vi "6009 LV71.vi"() -> ()   [LabVIEW 2020]
uses:
  <vilib>/DAQmx/read.llb/DAQmx Read.vi
  <vilib>/DAQmx/read.llb/DAQmx Read (Analog 1D Wfm NChan NSamp).vi
  <vilib>/DAQmx/miscellaneous.llb/DAQmx Fill In Error Info.vi
panel:
  in  "Channel B":tag
  in  "Channel A":tag
  out "error out":errorcluster
  out "Origin ref":refnum<k7>
  in  "Show Origin":bool
  out "path":path
  out "OriginWks":refnum<k7>
  out "Samples in Buffer\n(Scan Backlog)":u32
  out "Reading Fast\nEnough?":bool
  in  "Read Wait (ms)":i32=200
  in  "Sampling Rate (Hz)":dbl(slide)=1000.0 min=100.0 max=20000.0 step=100.0 scale=100.0..20000.0 scale format="%#_4f"
  out "Buffer Size":dbl=1000.0
  out "Waveforms":waveform(dbl)[](graph)
  in  "stop":bool
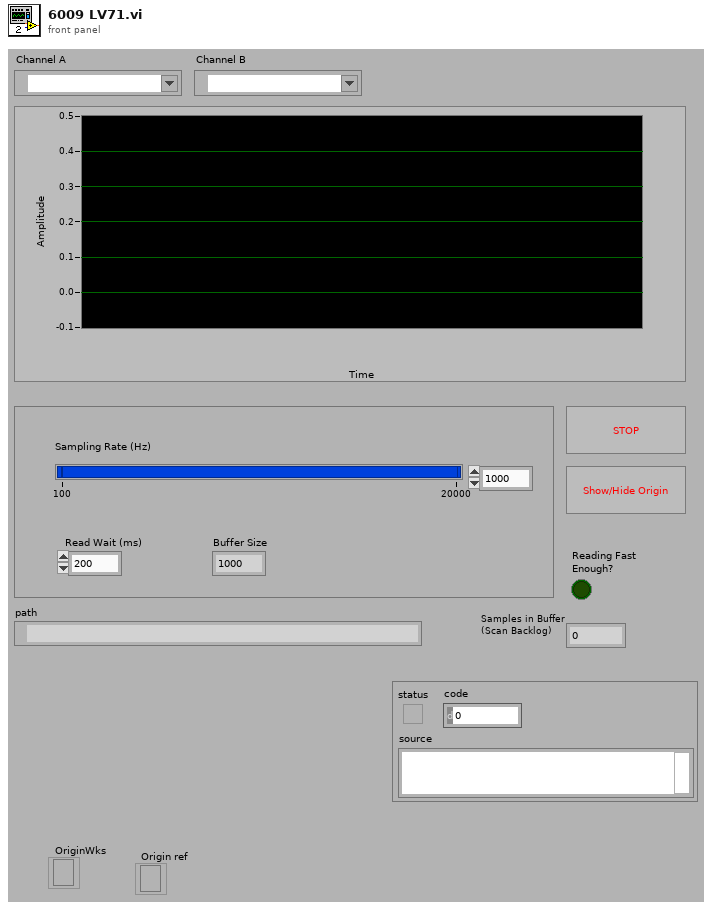
[diagram p1: front panel]
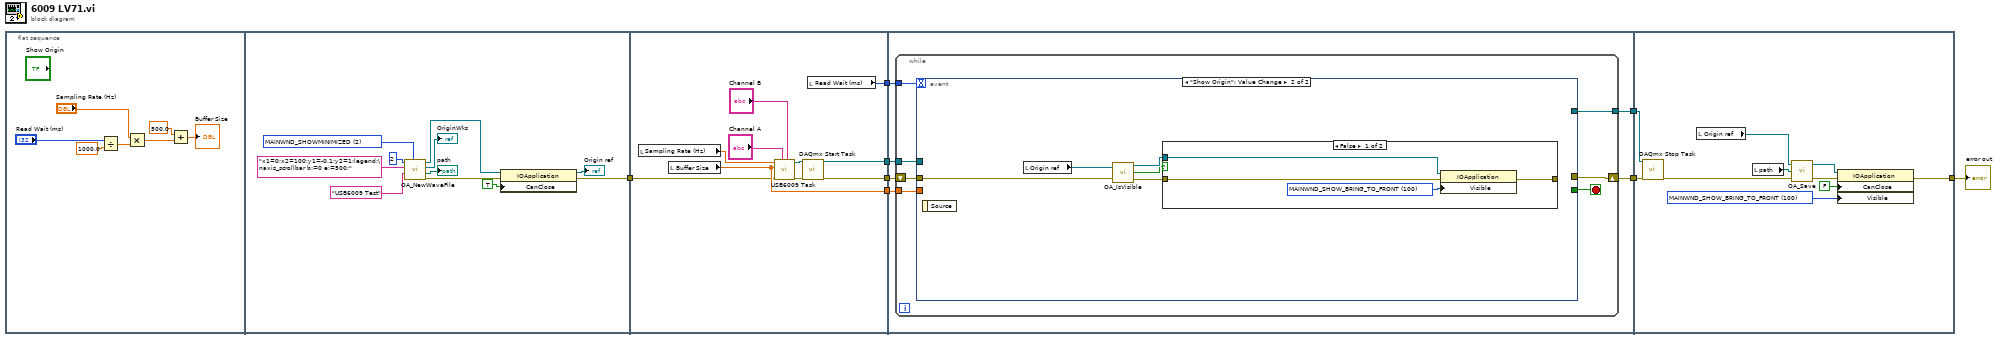
[diagram p0: block diagram]
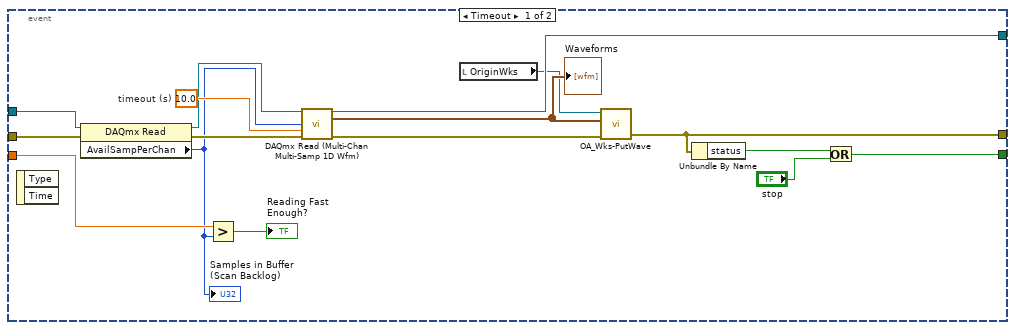
[diagram p2: hidden frame]
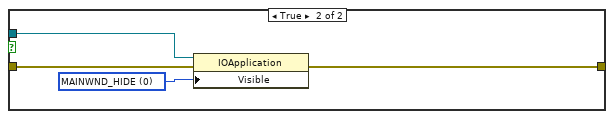
[diagram p3: hidden frame]
diagram:
  n1 = flat-sequence {
    tunnel: [w16] -> w2
    tunnel: [w33] -> w7
    tunnel: [w32] -> w6
    tunnel: [w31] -> w5
    tunnel: [w30] -> w4
    tunnel: w2 -> [w29]
    tunnel: [w42] -> w8
    tunnel: w7 -> [w39]
    tunnel: w6 -> [w41]
    tunnel: w5 -> [w40]
    tunnel: w4 -> [w38]
    tunnel: [w37] -> w3
    tunnel: w8 -> [w86]
    tunnel: w3 -> [w85]
    tunnel: [w79] -> w1
    frame #0 {
      n2 = Divide(x="Read Wait (ms)", y=1000.0 ("x")) -> (x/y=w12:dbl)
      n3 = Multiply(x="Sampling Rate (Hz)", y=w12) -> (x*y=w10:dbl)
      n4 = Add(x=500.0, y=w10) -> (x+y=→"Buffer Size":dbl)
    }
    frame #1 {
      w26 = 2 items=["MAINWND_HIDE"=0, "MAINWND_SHOW"=1, "MAINWND_SHOWMINIMIZED"=2, "MAINWND_SHOWMAXIMIZED"=3, "MAINWND_SHOW_BRING_TO_FRONT"=100] ("Visible")
      n5 = call "OA_NewWaveFile.vi"("Visible"=w26, "Origin file name"="USB6009 Test", "graph script"="x1=0;x2=100;y1=-0.1;y2=1;legend;\naxis_scrollbar b:=0 e:=500;", "number of columns"=2) -> ("error out"=w17:errorcluster, "path out"=→"path":path, "Origin.Worksheet"=→"OriginWks":refnum<k7>, "Origin.IOApplication"=w18:refnum<k7>)  [unwired: 4 in]
      n6 = property class="IOApplication"(reference=w18, error in=w17, "CanClose"=TRUE) -> (reference out=→"Origin ref":refnum<k7>, error out=w16:errorcluster)
    }
    frame #2 {
      n7 = local read "Sampling Rate (Hz)"() -> (w36:dbl)
      n8 = local read "Buffer Size"() -> (w31:dbl)
      n9 = call "USB6009 Task.vi"("physical channels 2"="Channel B", "physical channels"="Channel A", "error in"=w29, "rate"=w31, "number of samples"=w36) -> ("error out"=w35:errorcluster, "task out"=w34:refnum<k21>)  [unwired: 5 in]
      n10 = call <vilib>:"DAQmx Start Task.vi"("task/channels in"=w34, "error in"=w35) -> ("task out"=w32:refnum<k21>, "error out"=w33:errorcluster)  [unwired: 12 in]
      n11 = local read "Read Wait (ms)"() -> (w30:i32)
    }
    frame #3 {
      n12 = while {
        tunnel: [w49] -> w42
        tunnel: w41 -> [w48]
        tunnel: w40 -> [w47]
        shift-right: [w45] -> w37
        shift-left: w39 -> [w46]
        tunnel: w38 -> [w44]
        stop <- w43 stop-if-true
        n13 = event shown="[1] \"Show Origin\": Value Change" {
          selector: _ -> [_ _]
          dyn-events: _ -> [_ _]
          timeout: w44 -> [_ _]
          tunnel: [w65 _] -> w49
          tunnel: w48 -> [w64 _]
          tunnel: w47 -> [w63 _]
          tunnel: w46 -> [w52 w66]
          tunnel: [w50 _] -> w45
          tunnel: [w51 _] -> w43
          event Timeout {
            w60 = 10.0  # timeout (s)
            n14 = event-data() -> ()  [unwired: 1 in, 2 out]
            n15 = property class="DAQmx Read"(reference=w64, error in=w52) -> (reference out=w56:refnum<k21>, error out=w59:errorcluster, "AvailSampPerChan"=w58:u32)
            "Samples in Buffer\n(Scan Backlog)" <- w58
            n16 = Greater?(x=w63, y=w58) -> (0:→"Reading Fast\nEnough?":bool)
            n17 = call-poly "DAQmx Read (Multi-Chan Multi-Samp 1D Wfm).vi"("task/channels in"=w56, "number of samples per channel"=w58, "timeout"=w60, "error in"=w59) -> ("task out"=w65:refnum<k21>, "data"=w55:waveform(dbl)[], "error out"=w54:errorcluster)  [unwired: 9 in]
            "Waveforms" <- w55
            n18 = local read "OriginWks"() -> (w53:refnum<k7>)
            n19 = call "OA_Wks-PutWave.vi"("Origin.Worksheet"=w53, "Dynamic Data"=w55, "error in (no error)"=w54) -> ("error IO"=w50:errorcluster)  [unwired: 3 in, 1 out]
            n20 = Unbundle By Name(w50) -> ("status"=w62:bool)
            n21 = Or(x=w62, y="stop") -> (x .or. y?=w51:bool)
          }
          event "Show Origin": Value Change {
            n22 = event-data() -> ()  [unwired: 1 in, 1 out]
            n23 = local read "Origin ref"() -> (w67:refnum<k7>)
            n24 = call "OA_IsVisible.vi"("Origin.IOApplication"=w67, "Error IO"=w66) -> ("Origin.IOApplication 2"=w70:refnum<k7>, "IsVisible"=w68:bool, "error"=w69:errorcluster)
            n25 = case shown="False" w68 {
              tunnel: w70 -> [w73 w77]
              tunnel: w69 -> [w72 w76]
              tunnel: [w71 w75] -> _
              frame False {
                w74 = 100 items=["MAINWND_HIDE"=0, "MAINWND_SHOW"=1, "MAINWND_SHOWMINIMIZED"=2, "MAINWND_SHOWMAXIMIZED"=3, "MAINWND_SHOW_BRING_TO_FRONT"=100] ("Visible")
                n26 = property class="IOApplication"(reference=w73, error in=w72, "Visible"=w74) -> (error out=w71:errorcluster)  [unwired: 1 out]
              }
              frame True {
                w78 = 0 items=["MAINWND_HIDE"=0, "MAINWND_SHOW"=1, "MAINWND_SHOWMINIMIZED"=2, "MAINWND_SHOWMAXIMIZED"=3, "MAINWND_SHOW_BRING_TO_FRONT"=100] ("Visible")
                n27 = property class="IOApplication"(reference=w77, error in=w76, "Visible"=w78) -> (error out=w75:errorcluster)  [unwired: 1 out]
              }
            }
          }
        }
      }
    }
    frame #4 {
      w80 = 100 items=["MAINWND_HIDE"=0, "MAINWND_SHOW"=1, "MAINWND_SHOWMINIMIZED"=2, "MAINWND_SHOWMAXIMIZED"=3, "MAINWND_SHOW_BRING_TO_FRONT"=100] ("Visible")
      n28 = call <vilib>:"DAQmx Stop Task.vi"("task/channels in"=w86, "error in"=w85) -> ("error out"=w87:errorcluster)  [unwired: 12 in, 1 out]
      n29 = local read "Origin ref"() -> (w84:refnum<k7>)
      n30 = local read "path"() -> (w88:path)
      n31 = call "OA_Save.vi"("Error IO"=w87, "Path"=w88, "Origin.IOApplication"=w84) -> ("Error IO Out"=w81:errorcluster, "Origin.IOApplication"=w83:refnum<k7>)  [unwired: 1 out]
      n32 = property class="IOApplication"(reference=w83, error in=w81, "CanClose"=FALSE, "Visible"=w80) -> (error out=w79:errorcluster)  [unwired: 1 out]
    }
  }
  "error out" <- w1
